vi "station_name_selector.vi"(6 "station":T1, 8 "error_in":errorcluster) -> (0 "error_out":errorcluster, 2 "all_station_names":string[](array[string]), 3 "current_station_name":string)   [LabVIEW 2020]
uses:
  station.ctl
  FGV/main_ini/FGV_PROXY_config_info.ctl
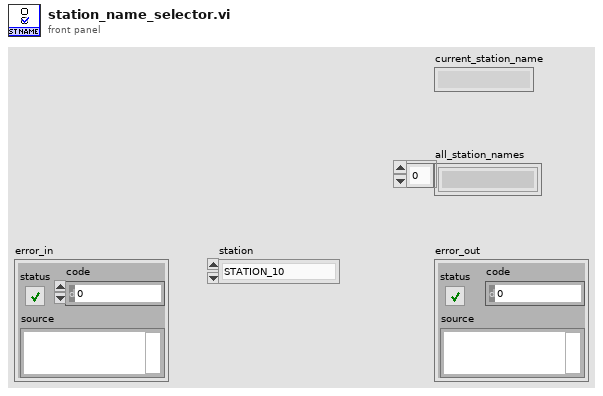
[diagram p1: front panel]
types:
  T1 = typedef "station.ctl" = enum16{"STATION_10", "STATION_20", "STATION_30", "STATION_40", "STATION_50", "STATION_60", "STATION_70", "STATION_80", "STATION_90", "STATION_100", "STATION_110", "STATION_120", "STATION_165", "MAIN"}
  T2 = typedef "FGV_PROXY_config_info.ctl" = enum16{"initialize", "set", "get"}
  T3 = typedef "PROXY_all_config_info.ctl" = cluster{"main_ini_file":T4, "SQL Password":string, "queue_refnums":T5, "number_of_stations":i32}
  T4 = typedef "PROXY_main_ini_file.ctl" = cluster{"SQL Driver":string, "SQL Server":string, "SQL Database":string, "SQL UID":string, "Reference table":string, "Reference history":string, "Archivisation CFG table":string, "Archivisation CFG history":string, "User table":string, "User history":string, "default language":string, "REF CHG listener IP":string, "REF CHG listener port":u16, "ST 10 name":string, "ST 10 listener IP":string, "ST 10 listener port":u16, "ST 20 name":string, "ST 20 listener IP":string, "ST 20 listener port":u16, "ST 30 name":string, "ST 30 listener IP":string, "ST 30 listener port":u16, "ST 40 name":string, "ST 40 listener IP":string, "ST 40 listener port":u16, "ST 50 name":string, "ST 50 listener IP":string, "ST 50 listener port":u16, "ST 60 name":string, "ST 60 listener IP":string, "ST 60 listener port":u16, "ST 70 name":string, "ST 70 listener IP":string, "ST 70 listener port":u16, "ST 80 name":string, "ST 80 listener IP":string, "ST 80 listener port":u16, "ST 90 name":string, "ST 90 listener IP":string, "ST 90 listener port":u16, "ST 100 name":string, "ST 100 listener IP":string, "ST 100 listener port":u16, "ST 110 name":string, "ST 110 listener IP":string, "ST 110 listener port":u16, "ST 120 name":string, "ST 120 listener IP":string, "ST 120 listener port":u16, "ST 165 name":string, "ST 165 listener IP":string, "ST 165 listener port":u16}
  T5 = typedef "PROXY_queue_refnums.ctl" = cluster{"ST_10_queue":refnum<queue>, "ST_20_queue":refnum<queue>, "ST_30_queue":refnum<queue>, "ST_40_queue":refnum<queue>, "ST_50_queue":refnum<queue>, "ST_60_queue":refnum<queue>, "ST_70_queue":refnum<queue>, "ST_80_queue":refnum<queue>, "ST_90_queue":refnum<queue>, "ST_100_queue":refnum<queue>, "ST_110_queue":refnum<queue>, "ST_120_queue":refnum<queue>, "ST_165_queue":refnum<queue>}
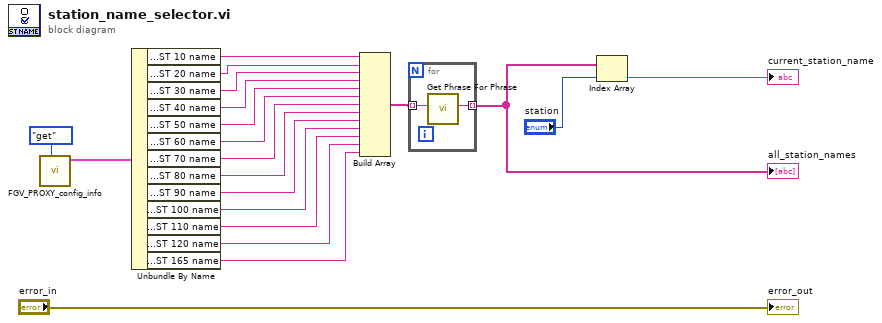
[diagram p0: block diagram]
diagram:
  n1 = call "FGV_PROXY_config_info.vi"("options"=FGV_PROXY_config_info."get") -> ("all_config_info_out"=w13:T3)  [unwired: 9 in, 1 out]
  n2 = Unbundle By Name(w13) -> ("main_ini_file.ST 10 name"=w20:string, "main_ini_file.ST 20 name"=w19:string, "main_ini_file.ST 30 name"=w18:string, "main_ini_file.ST 40 name"=w12:string, "main_ini_file.ST 50 name"=w11:string, "main_ini_file.ST 60 name"=w10:string, "main_ini_file.ST 70 name"=w9:string, "main_ini_file.ST 80 name"=w8:string, "main_ini_file.ST 90 name"=w7:string, "main_ini_file.ST 100 name"=w6:string, "main_ini_file.ST 110 name"=w5:string, "main_ini_file.ST 120 name"=w4:string, "main_ini_file.ST 165 name"=w3:string)
  n3 = Build Array(w20, w19, w18, w12, w11, w10, w9, w8, w7, w6, w5, w4, w3) -> (w2:string[])
  n4 = for {
    tunnel: w2 -> [w22] mode=indexing
    tunnel: [w21] -> w1 mode=indexing
    n5 = call "Get Phrase For Phrase.vi"("Phrase"=w22) -> ("Phrase"=w21:string)  [unwired: 9 in, 1 out]
  }
  "all_station_names" <- w1
  n6 = Index Array(array=w1, index="station") -> (element=→"current_station_name":string)
  "error_out" <- "error_in"
